vi "GetPositions.vi"(8 "error in (no error)":errorcluster, 11 "MotorController in":refnum<class "MotorController.lvclass">) -> (0 "error out":errorcluster, 3 "MotorController out":refnum<class "MotorController.lvclass">, 4 "Stage Position":u16, 5 "Polarizer 2 Position":u16, 6 "Sample Position":u16, 7 "Polarizer 1 Position":u16)   [LabVIEW 2019, in "MotorController.lvclass"]
uses:
  MotorController.lvclass
  MotorController.lvclass/MotorController.ctl
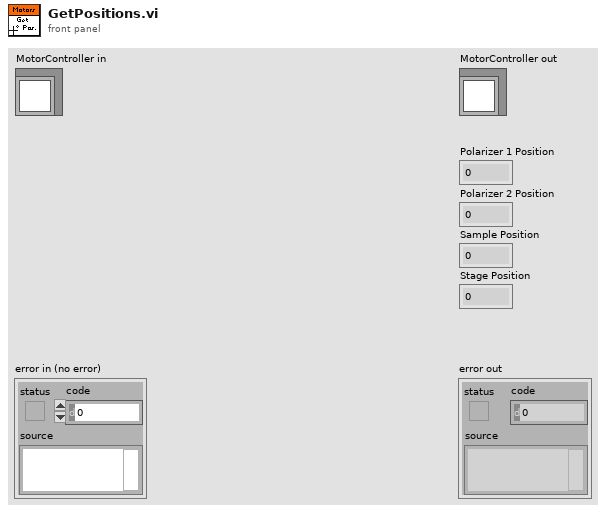
[diagram p1: front panel]
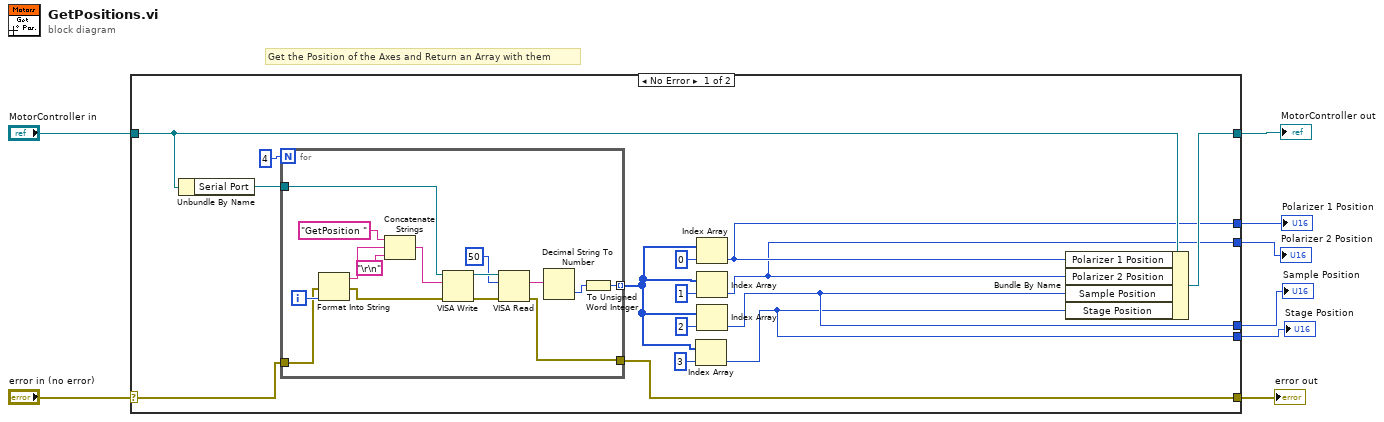
[diagram p0: block diagram]
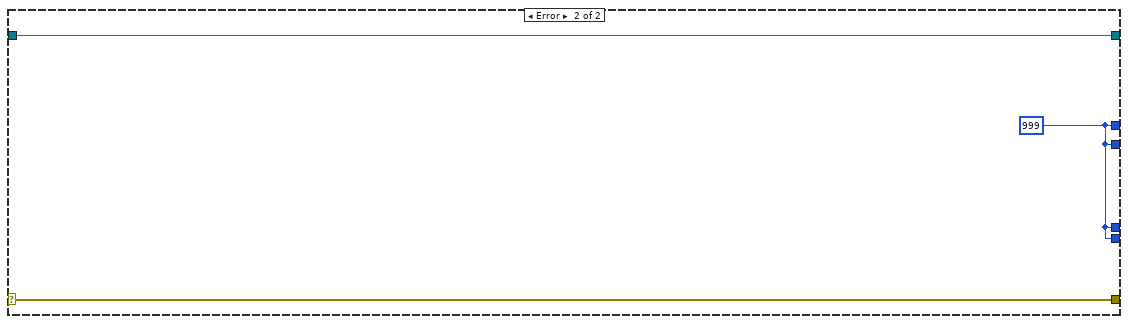
[diagram p2: hidden frame]
diagram:
  # "Get the Position of the Axes and Return an Array with them"
  n1 = case shown="No Error" "error in (no error)" {
    selector: "error in (no error)" -> [w22 w41]
    tunnel: [w20 w41] -> w7
    tunnel: [w13 w40] -> w5
    tunnel: "MotorController in" -> [w14 w40]
    tunnel: [w12 w39] -> w4
    tunnel: [w11 w39] -> w3
    tunnel: [w10 w39] -> w2
    tunnel: [w9 w39] -> w1
    frame No Error {
      n2 = Unbundle By Name(w14) -> ("Serial Port"=w21:refnum<visa-resource-name>)
      n3 = for {
        N: 4 -> [_]
        tunnel: w22 -> [w34]
        tunnel: w21 -> [w31]
        tunnel: [w25] -> w15 mode=indexing
        tunnel: [w24] -> w20
        i -> [w36]
        n4 = Format Into String(error in=w34, w36) -> (resulting string=w35:string, error out=w33:errorcluster)  [unwired: 2 in]
        n5 = Concatenate Strings("GetPosition ", w35, "\r\n") -> (w32:string)
        n6 = VISA Write(VISA resource name=w31, write buffer=w32, error in (no error)=w33) -> (VISA resource name out=w29:refnum<visa-resource-name>, error out=w30:errorcluster)  [unwired: 1 out]
        n7 = VISA Read(VISA resource name=w29, byte count=u32 50, error in (no error)=w30) -> (read buffer=w27:string, error out=w24:errorcluster)  [unwired: 2 out]
        n8 = Decimal String To Number(string=w27) -> (number=w26:i32)  [unwired: 2 in, 1 out]
        n9 = To Unsigned Word Integer(number=w26) -> (unsigned 16bit integer=w25:u16)
      }
      n10 = Index Array(array=w15, index=3) -> (element=w9:u16)
      n11 = Index Array(array=w15, index=0) -> (element=w12:u16)
      n12 = Index Array(array=w15, index=1) -> (element=w11:u16)
      n13 = Index Array(array=w15, index=2) -> (element=w10:u16)
      n14 = Bundle By Name(cluster=w14, "Polarizer 1 Position"=w12, "Polarizer 2 Position"=w11, "Sample Position"=w10, "Stage Position"=w9) -> (w13:refnum<class "MotorController.lvclass">)
    }
    frame Error {
      w39 = u16 999
    }
  }
  "error out" <- w7
  "MotorController out" <- w5
  "Polarizer 1 Position" <- w4
  "Polarizer 2 Position" <- w3
  "Sample Position" <- w2
  "Stage Position" <- w1
